vi "viewSensorData.vi"(8 "error in (no error)":errorcluster, 11 "TEI9150 in":refnum<class "Tovey9150.lvclass">) -> (0 "error out":errorcluster, 2 "Stored Sensor Data":string, 3 "TEI9150 out":refnum<class "Tovey9150.lvclass">)   [LabVIEW 2015]
uses:
  <userlib>/Common/SerialProtocols/SerialCommunicator/SerialCommunicator.lvclass
  Tovey9150.lvclass
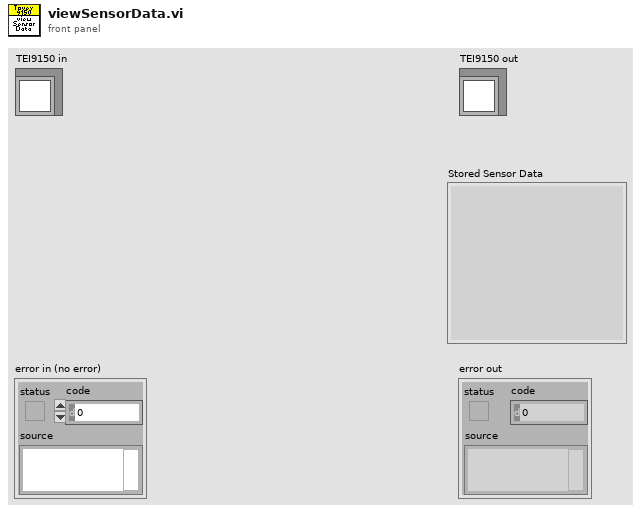
[diagram p1: front panel]
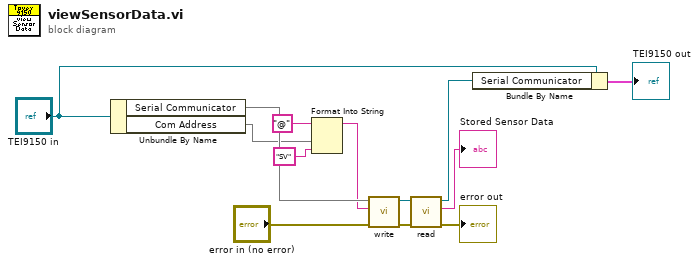
[diagram p0: block diagram]
diagram:
  n1 = Unbundle By Name("TEI9150 in") -> ("Serial Communicator"=w11, "Com Address"=w9)
  n2 = Format Into String(initial string="@", w9, "SV" ("input 2")) -> (resulting string=w7:string)  [unwired: 2 in, 1 out]
  n3 = call-dynamic "write.vi"("error in (no error)"="error in (no error)", "writeString"=w7, "SerialCommunicator in"=w11) -> ("error out"=w12:errorcluster, "SerialCommunicator out"=w13:refnum<class "SerialCommunicator.lvclass">)  [unwired: 7 in]
  n4 = call-dynamic "read.vi"("error in (no error)"=w12, "SerialCommunicator in"=w13) -> ("error out"=→"error out":errorcluster, "stringRead"=→"Stored Sensor Data":string, "SerialCommunicator out"=w3:refnum<class "SerialCommunicator.lvclass">)  [unwired: 7 in]
  n5 = Bundle By Name(cluster="TEI9150 in", "Serial Communicator"=w3) -> (→"TEI9150 out":cluster{})
